vi "Curtin1_Recalc.vi"(9 "Instrument:Test Name":string, 10 "Settings":T1={"Name of test"="", "Date"=timestamp(0 s since 1904-01-01), "Location"="", "Template"="", "Soundcard"="", "resolution"=32, "Sampling rate"=48000, "Ch1 Gain "=25.0, "Ch2 Gain"=10.0, "Sample time (s)"=0.3, "Pre-trigger (s)"=0.01, "Hammer Threshold"=10.0, "Positions"=12, "Taps/Position"=5, "Set Names"="", "Freq resolution"=10.0, "Hammer cutoff"=0.0, "Mic cutoff"=0.0, "Double bounce "=0.0, "Hammer Cal"=1.0, "dB Offset"=0.0, "Accel Cal"=1.0, "Vibrometer Cal"=1.0, "Mic Cal"=1.0, "Output"=2, "Voltage Cal"=1.0, "Vibrometer Port"="ASRL27::INSTR", "Range"=50, "High Pass"=2, "Bandwidth"=25, "X Range"=[], "Y Range"=[], "dB Spread"=0.0, "Trigger"=0, "Ch_1"=1, "Ch_2"=2, "flip?"=FALSE, "60Hz"=FALSE, "Time offset"=0.0, "Piezo Cal"=1.0, "Default Notes"=""} {"Ch_2" min=1 step=1; "Ch_1" min=1 max=100 step=1; "Trigger" items=["Hammer (force)", "Self-tap", "Spacebar"]; "Bandwidth" items=["1 kHz"=1, "5 kHz"=5, "10 kHz"=10, "25 kHz"=25, "50 kHz"=50, "100 kHz"=100]; "High Pass" items=["Off", "13 Hz", "104 Hz"]; "Range" items=["10 mm/s"=1, "20 mm/s"=2, "50 mm/s"=5, "100 mm/s"=10, "200 mm/s"=20, "500 mm/s"=50, "1 m/s"=100, "2 m/s"=200]; "Output" items=["Accelerometer", "Speed (from acceleration)", "Microphone", "Vibrometer", "Piezo"]; "Voltage Cal" format="%#_13g"; "Ch2 Gain" format="%#_13g"; "Ch1 Gain" format="%#_13g"; "Double bounce" min=0.0; "Mic cutoff" min=0.0 format="%#_4g"; "Hammer cutoff" min=0.0 format="%#_4g"; "Freq resolution" min=0.0; "Pre-trigger (s)" format="%#_13g"; "Date" format="%<%H:%M\n%d/%m/%y>T"; "resolution" items=["16 bit"=16, "24 bit"=24, "32 bit"=32]; "Sampling rate" items=["22050 samp/s"=22050, "44100 samp/s"=44100, "48000 samp/s"=48000]}, 11 "Path To Raw Folder":path) -> ()   [LabVIEW 2022 SP3]
uses:
  PreferencesControl.ctl
panel:
  in  "Abort":bool
  out "size(s)":i32
  out "Hammer Spectra":cluster{dbl, "df":dbl, "FFT {X}":dbl[]}[](graph)
  out "Microphone Spectra":cluster{dbl, "df":dbl, "FFT {X}":dbl[]}[](graph)
  out "Average FRF":cluster{dbl, "df":dbl, dbl[]}[](graph)
  out "Hammer":cluster{dbl, "dt":dbl, "Y":dbl[]}[](graph)
  out "Microphone":cluster{dbl, "dt":dbl, "Y":dbl[]}[](graph)
  out "Progress Bar":picture
  out "Last Path":path
  # "Hz"
  # "dB"
  # "dB"
  # "sec"
  # "sec"
  # "mV/Pa"
  # "mV/m/s2"
  # "mV/mm/s"
  # "V/N"
  # "sec"
  # "sec"
  # "mV/N"
  # "a.u."
  # "a.u."
  # "sec"
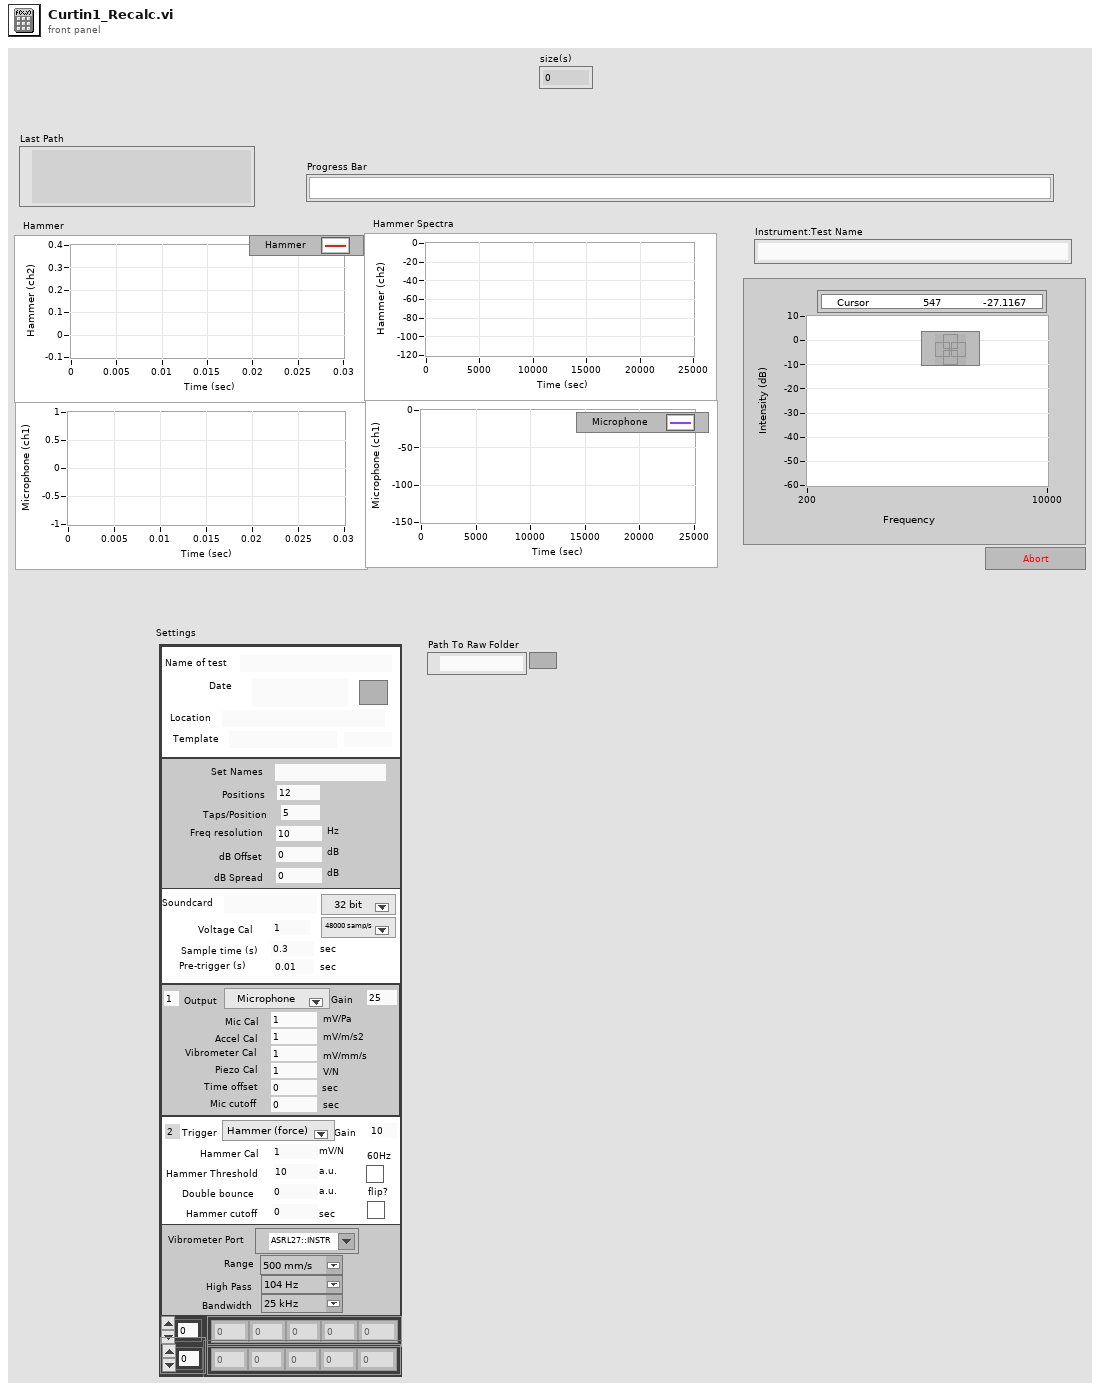
[diagram p1: front panel]
types:
  T1 = typedef "PreferencesControl.ctl" = cluster{"Name of test":string, "Date":timestamp, "Location":string, "Template":string, "Soundcard":string, "resolution":u16, "Sampling rate":u16, "Ch1 Gain ":dbl, "Ch2 Gain":dbl, "Sample time (s)":dbl, "Pre-trigger (s)":dbl, "Hammer Threshold":dbl, "Positions":i16, "Taps/Position":i16, "Set Names":string, "Freq resolution":dbl, "Hammer cutoff":dbl, "Mic cutoff":dbl, "Double bounce ":dbl, "Hammer Cal":dbl, "dB Offset":dbl, "Accel Cal":dbl, "Vibrometer Cal":dbl, "Mic Cal":dbl, "Output":u16, "Voltage Cal":dbl, "Vibrometer Port":refnum<visa-resource-name>, "Range":u16, "High Pass":u16, "Bandwidth":u16, "X Range":cluster{"Minimum":dbl, "Maximum":dbl, "Increment":dbl, "Minor Increment":dbl, "Start":dbl}[], "Y Range":cluster{"Minimum":dbl, "Maximum":dbl, "Increment":dbl, "Minor Increment":dbl, "Start":dbl}[], "dB Spread":dbl, "Trigger":u16, "Ch_1":u8, "Ch_2":u8, "flip?":bool, "60Hz":bool, "Time offset":dbl, "Piezo Cal":dbl, "Default Notes":string}
  T2 = typedef "LVBoundsTypeDef.ctl" = cluster{"Width":u32, "Height":u32}
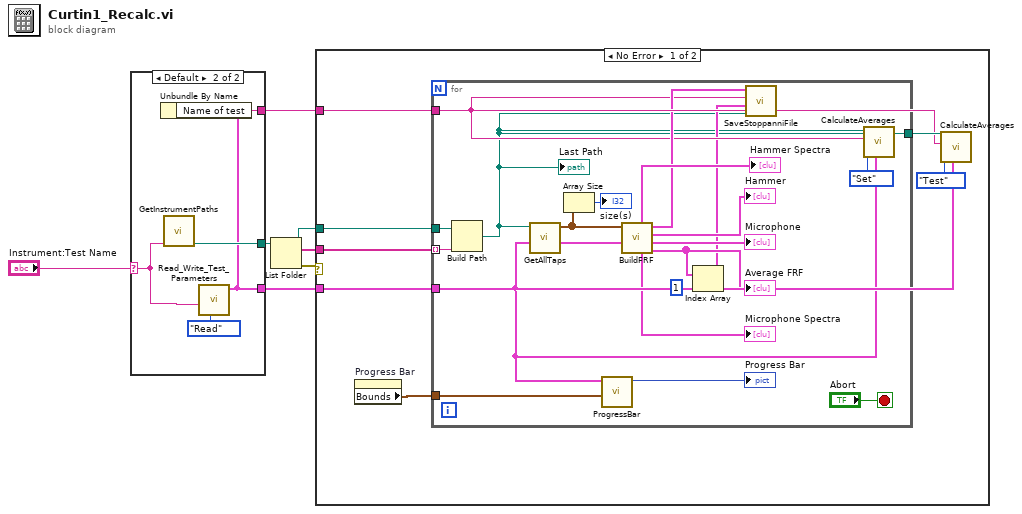
[diagram p0: block diagram]
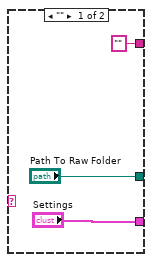
[diagram p2: hidden frame]
diagram:
  n1 = case shown="Default" "Instrument:Test Name" {
    selector: "Instrument:Test Name" -> [_ w11]
    tunnel: ["Settings" w13] -> w4
    tunnel: ["Path To Raw Folder" w14] -> w3
    tunnel: ["" ("Name of test") w12] -> w1
    frame "" {
    }
    frame Default {
      n2 = call "GetInstrumentPaths.vi"("Instrument"=w11) -> ("Path To Raw Folder"=w14:path)  [unwired: 6 in, 4 out]
      n3 = call "Read_Write_Test_Parameters.vi"("Task"=enum16{"Save", "Read", "Clear"}."Read", "Instrument Name"=w11) -> ("Settings"=w13:T1)  [unwired: 8 in, 1 out]
      n4 = Unbundle By Name(w13) -> ("Name of test"=w12:string)
    }
  }
  n5 = List Folder(path=w3) -> (path out=w6:path, filenames=w7:string[], error out=w5:errorcluster)  [unwired: 3 in, 1 out]
  n6 = case shown="No Error" w5 {
    tunnel: w7 -> [w22 _]
    tunnel: w6 -> [w21 _]
    tunnel: w4 -> [w17 _]
    tunnel: w1 -> [w16 _]
    frame No Error {
      n7 = property on="Progress Bar" class="Pict"() -> ("Bounds"=w18:T2)  [unwired: 2 in, 2 out]
      n8 = for {
        tunnel: w22 -> [w41] mode=indexing
        tunnel: w21 -> [w40]
        tunnel: w17 -> [w24]
        tunnel: [w23] -> w19
        tunnel: w16 -> [w30]
        tunnel: w18 -> [w25]
        stop <- "Abort" stop-if-true
        n9 = Build Path(base path=w40, name or relative path=w41) -> (appended path=w23:path)
        "Last Path" <- w23
        n10 = call "GetAllTaps.vi"("Last Path"=w23) -> ("taps in pos"=w38:waveform(dbl)[])  [unwired: 8 in, 2 out]
        n11 = Array Size(array=w38) -> (size(s)=→"size(s)":i32)
        n12 = call "ProgressBar.vi"("Bounds"=w25, "Settings"=w24) -> ("Progress Bar"=→"Progress Bar":picture)  [unwired: 7 in, 2 out]
        n13 = call "BuildFRF.vi"("Settings"=w24, "Data In"=w38) -> ("Average FRF"=w27:cluster{dbl, "df":dbl, dbl[]}[], "Microphone"=→"Microphone":cluster{dbl, "dt":dbl, "Y":dbl[]}[], "Hammer"=→"Hammer":cluster{dbl, "dt":dbl, "Y":dbl[]}[], "Complex FRF"=w32:cluster{"t0":dbl, "dt":dbl, "Y":cdb[]}, "Microphone Spectra"=→"Microphone Spectra":cluster{"x0":dbl, "df":dbl, dbl[]}[], "Hammer Spectra"=→"Hammer Spectra":cluster{dbl, "df":dbl, "FFT {X}":dbl[]}[])  [unwired: 4 in]
        "Average FRF" <- w27
        n14 = Index Array(array=w27, index=1) -> (element=w26:cluster{dbl, "df":dbl, dbl[]})
        n15 = call "SaveStoppanniFile.vi"("Last Path"=w23, "Coherence in"=w26, "Inst:Test Name"=w30, "Complex FRF"=w32) -> ()  [unwired: 7 in, 1 out]
        n16 = call "CalculateAverages.vi"("Settings"=w24, "Task"=enum16{"Set", "Test"}."Set", "Inst:Test Name"=w30, "Last Data File"=w23) -> ()  [unwired: 8 in]
      }
      n17 = call "CalculateAverages.vi"("Settings"=w17, "Task"=enum16{"Set", "Test"}."Test", "Inst:Test Name"=w16, "Last Data File"=w19) -> ()  [unwired: 8 in]
    }
    frame Error {
    }
  }
